vi "TopLeftRightBottomArrays.vi"(8 "error in (no error)":errorcluster, 11 "PentaPanesGUI in":refnum<class "PentaPanes.lvclass">) -> (0 "error out":errorcluster, 1 "Pane Position numbers":T1[](array[typedef]) items=["Top", "Left", "Center", "Right", "Bottom"], 2 "Splitters":refnum<vi>[](array[refnum]), 3 "PentaPanesGUI out":refnum<class "PentaPanes.lvclass">, 4 "Pane position Strings":string[](array[string]), 5 "Panes":refnum<vi>[](array[refnum]), 6 "Top/Left/Right/Bottom arrays":T2 {"Position Integer" items=["Top", "Left", "Center", "Right", "Bottom"]})   [LabVIEW 2022 SP3, in "PentaPanesLibrary.lvlib" / "PentaPanes.lvclass"]
uses:
  PentaPanes.lvclass
  PanePosition.ctl
  TopLeftRightBottomArrays.ctl
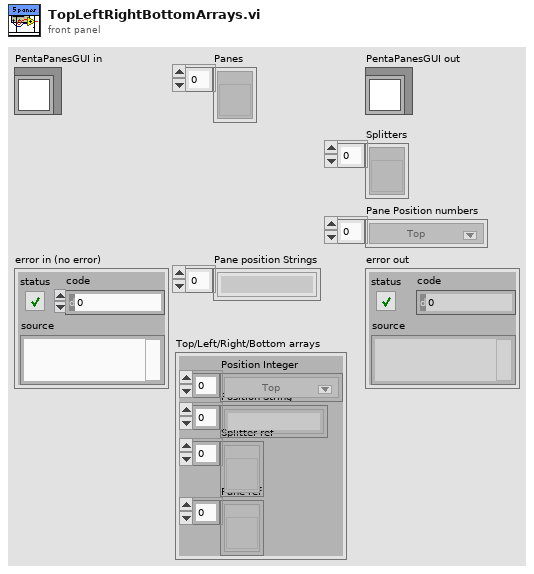
[diagram p1: front panel]
types:
  T1 = typedef "PentaPanesLibrary.lvlib/PentaPanes.lvclass/PanePosition.ctl" = u16
  T2 = cluster{"Position Integer":T1[], "Position String":string[], "Splitter ref":refnum<vi>[], "Pane ref":refnum<vi>[]}
  T3 = typedef "PentaPanesLibrary.lvlib/PentaPanes.lvclass/TopLeftRightBottomArrays.ctl" = cluster{"Position Integer":T1[], "Position String":string[], "Splitter ref":refnum<vi>[], "Pane ref":refnum<vi>[]}
  T4 = cluster{T1[], string[], refnum<vi>[], refnum<vi>[]}
  T5 = typedef "PentaPanesLibrary.lvlib/PentaPanes.lvclass/SplittersCluster.ctl" = cluster{"Top Splitter":refnum<vi>, "Left Splitter":refnum<vi>, "Right Splitter":refnum<vi>, "Bottom Splitter":refnum<vi>}
  T6 = typedef "PentaPanesLibrary.lvlib/PentaPanes.lvclass/PanesCluster.ctl" = cluster{"Top Pane":refnum<vi>, "Left Pane":refnum<vi>, "Center Pane":refnum<vi>, "Right Pane":refnum<vi>, "Bottom Pane":refnum<vi>}
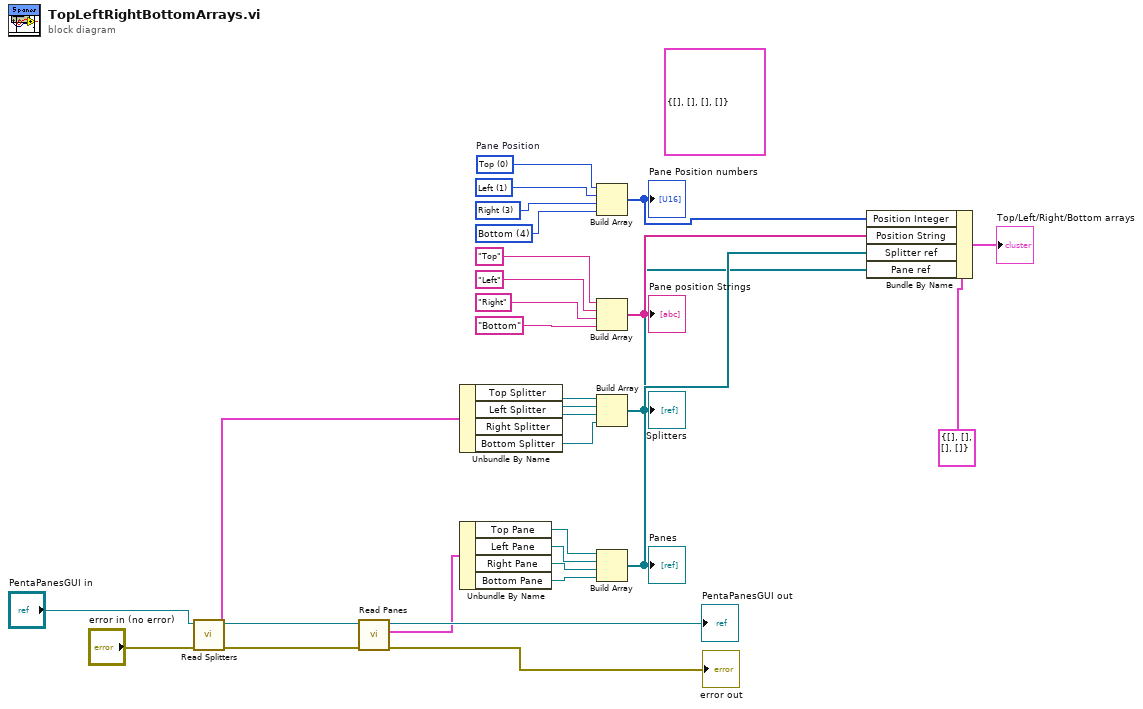
[diagram p0: block diagram]
diagram:
  (unwired) T4 {[], [], [], []} ("output cluster")
  w15 = T1 4 items=["Top", "Left", "Center", "Right", "Bottom"] ("Pane Position")
  w14 = T1 3 items=["Top", "Left", "Center", "Right", "Bottom"] ("Pane Position")
  w13 = T1 1 items=["Top", "Left", "Center", "Right", "Bottom"] ("Pane Position")
  w12 = T1 0 items=["Top", "Left", "Center", "Right", "Bottom"]  # Pane Position
  n1 = call-dynamic "Read Splitters.vi"("error in (no error)"="error in (no error)", "PentaPanesGUI in"="PentaPanesGUI in") -> ("error out"=w25:errorcluster, "Splitters"=w8:T5, "PentaPanesGUI out"=w18:refnum<class "PentaPanes.lvclass">)  [unwired: 7 in]
  n2 = call-dynamic "Read Panes.vi"("error in (no error)"=w25, "PentaPanesGUI in"=w18) -> ("error out"=→"error out":errorcluster, "Panes"=w19:T6, "PentaPanesGUI out"=→"PentaPanesGUI out":refnum<class "PentaPanes.lvclass">)  [unwired: 7 in]
  n3 = Unbundle By Name(w8) -> ("Top Splitter"=w9:refnum<vi>, "Left Splitter"=w10:refnum<vi>, "Right Splitter"=w11:refnum<vi>, "Bottom Splitter"=w17:refnum<vi>)
  n4 = Unbundle By Name(w19) -> ("Top Pane"=w21:refnum<vi>, "Left Pane"=w22:refnum<vi>, "Right Pane"=w23:refnum<vi>, "Bottom Pane"=w24:refnum<vi>)
  n5 = Build Array(w12, w13, w14, w15) -> (w5:T1[])
  "Pane Position numbers" <- w5
  n6 = Build Array("Top", "Left", "Right", "Bottom") -> (w4:string[])
  "Pane position Strings" <- w4
  n7 = Build Array(w9, w10, w11, w17) -> (w3:refnum<vi>[])
  "Splitters" <- w3
  n8 = Build Array(w21, w22, w23, w24) -> (w2:refnum<vi>[])
  "Panes" <- w2
  n9 = Bundle By Name(cluster=T3 {"Position Integer"=[], "Position String"=[], "Splitter ref"=[], "Pane ref"=[]} ("Top/Left/Right/Bottom arrays"), "Position Integer"=w5, "Position String"=w4, "Splitter ref"=w3, "Pane ref"=w2) -> (→"Top/Left/Right/Bottom arrays":T3)
